vi "setOffset.vi"(8 "error in (no error)":errorcluster, 10 "Offset":dbl, 11 "AnalogOutput.lvclass in":refnum<class "AnalogOutput.lvclass">) -> (0 "error out":errorcluster, 3 "AnalogOutput.lvclass out":refnum<class "AnalogOutput.lvclass">)   [LabVIEW 2009, in "Hardware.lvlib" / "Channels.lvlib" / "AnalogOutput.lvclass"]
uses:
  AnalogOutput.lvclass
  AnalogOutput.lvclass/AnalogOutput.ctl
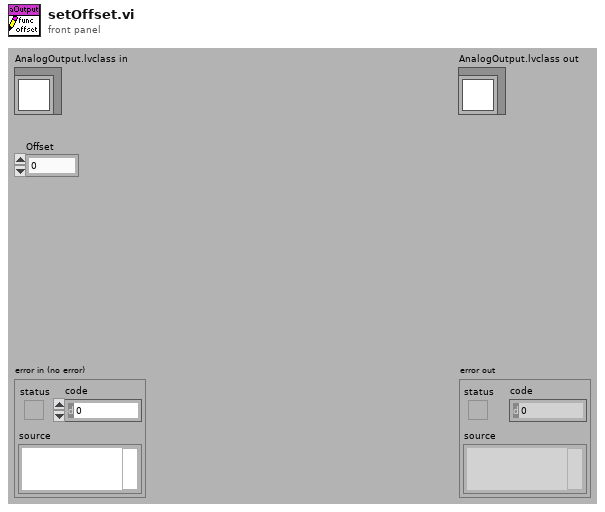
[diagram p1: front panel]
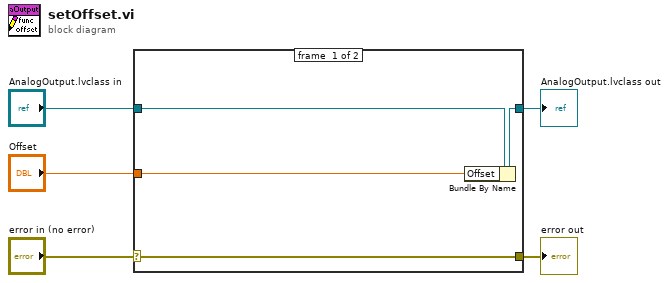
[diagram p0: block diagram]
diagram:
  n1 = case shown="No Error" "error in (no error)" {
    selector: "error in (no error)" -> [w9 w10]
    tunnel: [w9 w10] -> w4
    tunnel: [w7 w11] -> w2
    tunnel: "AnalogOutput.lvclass in" -> [w8 w11]
    tunnel: "Offset" -> [w6 _]
    frame #0 {
      n2 = Bundle By Name(cluster=w8, "Offset"=w6) -> (w7:refnum<class "AnalogOutput.lvclass">)
    }
    frame #1 {
    }
  }
  "error out" <- w4
  "AnalogOutput.lvclass out" <- w2
